vi "Wait Until Cancelled or Complete.vi"(6 "done channel":T1, 8 "error in (no error)":errorcluster, 9 "ms polling interval":i64=1, 10 "scope session":refnum<k15>, 11 "measure call context in":refnum<class "Measure Call Context.lvclass">) -> (0 "error out":errorcluster, 3 "neasure call context out":refnum<class "Measure Call Context.lvclass">)   [LabVIEW 2021, in "NIScopeAcquireWaveform.lvlib"]
uses:
  NIScopeAcquireWaveform.lvlib
  <extravilib>/ChannelInstances/One Element Stream-bool/)Channel.ctl
  <vilib>/Plug-In SDKs/Measurements/Measure Call Context/Measure Call Context.lvclass
  <vilib>/Platform/TimedLoop/XDataNode/timing_clust.ctl
  <vilib>/Platform/TimedLoop/XDataNode/nitl_modes.ctl
  <vilib>/Platform/TimedLoop/XDataNode/wakeup.ctl
  <extravilib>/ChannelInstances/One Element Stream-bool/Read With Abort.vi
  <extravilib>/ChannelInstances/One Element Stream-bool/EndpointRead.vi
  <vilib>/platform/TimedLoop/XDataNode/XDataNode.xnode
  <vilib>/Platform/TimedLoop/XDataNode/XDNodeRunTimeDep.lvlib
  <extravilib>/ChannelInstances/One Element Stream-bool.lvlib
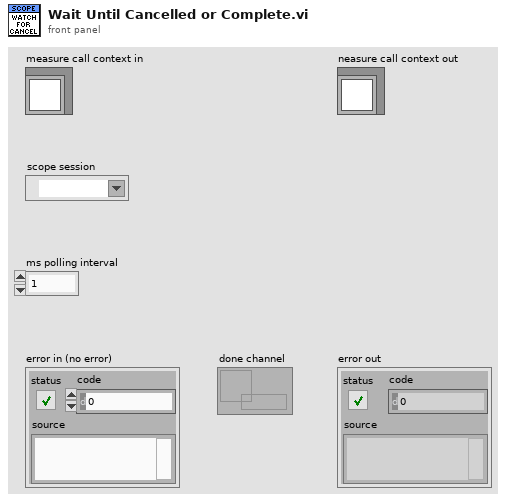
[diagram p1: front panel]
types:
  T1 = typedef "One Element Stream-bool.lvlib/)Channel.ctl" = refnum<queue>
  T2 = typedef "XDNodeRunTimeDep.lvlib/timing_clust.ctl" = cluster{"Expected End [f-1]":u64, "Actual End [f-1]":u64, "Finished Late? [f-1]":bool, "Expected End [i-1]":u64, "Actual End [i-1]":u64, "Finished Late? [i-1]":bool, "Expected Start [i]":u64, "Actual Start [i]":u64, "Expected Start [f]":u64, "Actual Start [f]":u64, "Source Name":string, "Structure Name":string, "Period":i64, "Deadline":i64, "Offset":i64, "Start":i64, "Priority":i32, "Timeout":i32, "Mode":T3, "Wakeup Reason":T4, "Error":errorcluster, "Source Type":string, "Secondary Source Type":string, "Global End Time":u64, "Global Start Time":u64, "Frame Duration":u64, "Iteration Duration":u64, "Assigned CPU":i32, "I/O Scan Engine Mode":u32}
  T3 = typedef "XDNodeRunTimeDep.lvlib/nitl_modes.ctl" = enum32{"No Change", "Process missed periods, maintain original phase", "Discard missed periods, maintain original phase", "Process missed periods, ignore original phase", "Discard missed periods, ignore original phase"}
  T4 = typedef "XDNodeRunTimeDep.lvlib/wakeup.ctl" = enum32{"Normal", "Aborted", "Asynchronous wakeup", "Timing source error", "Timed loop error", "Timeout"}
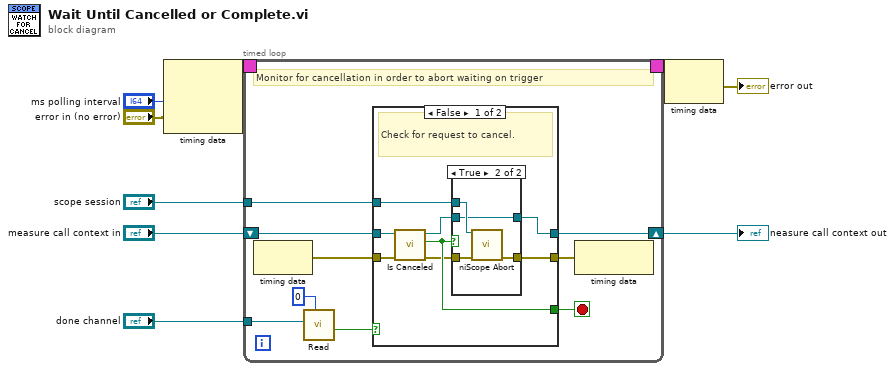
[diagram p0: block diagram]
diagram:
  n1 = node-c288("ms polling interval", "error in (no error)") -> (w9:T2)  [unwired: 1 in]
  n2 = timed-loop {
    tunnel: "scope session" -> [w16]
    timing: w9 -> [_]
    timing-out: [_] -> w8
    shift-right: [w17] -> w4
    shift-left: "measure call context in" -> [w18]
    tunnel: "done channel" -> [w11]
    stop <- w15 stop-if-true
    # "Monitor for cancellation in order to abort waiting on trigger"
    n3 = node-c288() -> (w14:errorcluster)  [unwired: 1 in]
    n4 = call <extravilib>:"Read.vi"("timeout in ms (-1)"=0, "channel"=w11) -> ("last element?"=w10:bool)  [unwired: 6 in, 3 out]
    n5 = case shown="False" w10 {
      selector: w10 -> [_ w35]
      tunnel: w18 -> [w26 w33]
      tunnel: [w25 w33] -> w17
      tunnel: w16 -> [w24 _]
      tunnel: [w23 w35] -> w15
      tunnel: w14 -> [w22 w34]
      tunnel: [w21 w34] -> w13
      frame False {
        # "Check for request to cancel."
        n6 = call <vilib>:"Is Canceled.vi"("error in"=w22, "measure call context in"=w26) -> ("error out"=w20:errorcluster, "is canceled?"=w23:bool, "measure call context out"=w19:refnum<class "Measure Call Context.lvclass">)  [unwired: 7 in]
        n7 = case shown="True" w23 {
          tunnel: w20 -> [w28 w32]
          tunnel: w19 -> [w27 w29]
          tunnel: [w28 w31] -> w21
          tunnel: [w27 w29] -> w25
          tunnel: w24 -> [_ w30]
          frame False {
          }
          frame True {
            n8 = call <instrlib>:"niScope Abort.vi"("instrument handle"=w30, "error in"=w32) -> ("error out"=w31:errorcluster)  [unwired: 12 in, 1 out]
          }
        }
      }
      frame True {
        # "Call completed normally without a request to cancel."
      }
    }
    n9 = node-c288(w13) -> ()  [unwired: 1 out]
  }
  "neasure call context out" <- w4
  n10 = node-c288(w8) -> (→"error out":errorcluster)
